vi "Interpret_LiDAR_Packet_Header.vi"(11 "Data in":u8[](array[numeric])) -> (2 "output cluster":T1 {"Ray Header Data"."Return Data Array"."Reflectance" format="%.6f %"; "Ray Header Data"."Return Data Array"."Range" format="%.4f M"; "Ray Header Data"."Return Data Array"."Existence Probability" format="%.4f %"; "Ray Header Data"."Elevation" format="%.6f"; "Ray Header Data"."Azimuth" format="%.6f"}, 3 "Remaining Data out":u8[](array[numeric]))   [LabVIEW 2018, in "LiDAR.lvlib" / "LiDAR.lvclass"]
uses:
  LiDAR.lvclass
  Controls/cls_Point_Cloud_Data.ctl
  Controls/cls_Point_Cloud_Packet_Header.ctl
  Controls/cls_Point_Cloud_Ray_Header.ctl
  Controls/cls_Point_Cloud_Return_Data.ctl
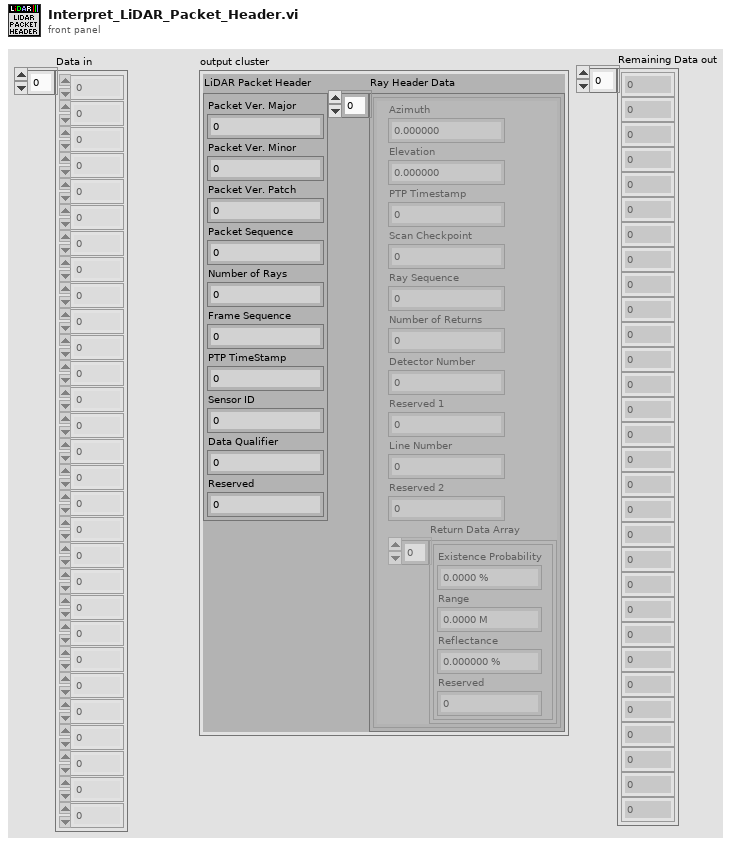
[diagram p1: front panel]
types:
  T1 = typedef "LiDAR.lvlib/LiDAR.lvclass/cls_Point_Cloud_Data.ctl" = cluster{"LiDAR Packet Header":T2, "Ray Header Data":T3[]}
  T2 = typedef "LiDAR.lvlib/LiDAR.lvclass/cls_Point_Cloud_Packet_Header.ctl" = cluster{"Packet Ver. Major":u8, "Packet Ver. Minor":u8, "Packet Ver. Patch":u8, "Packet Sequence":u8, "Number of Rays":u8, "Frame Sequence":u8, "PTP TimeStamp":u64, "Sensor ID":u8, "Data Qualifier":u8, "Reserved":u16}
  T3 = typedef "LiDAR.lvlib/LiDAR.lvclass/cls_Point_Cloud_Ray_Header.ctl" = cluster{"Azimuth":dbl, "Elevation":dbl, "PTP Timestamp":u32, "Scan Checkpoint":u8, "Ray Sequence":u8, "Number of Returns":u8, "Detector Number":u8, "Reserved 1":u8, "Line Number":u16, "Reserved 2":u32, "Return Data Array":T4[]}
  T4 = typedef "LiDAR.lvlib/LiDAR.lvclass/cls_Point_Cloud_Return_Data.ctl" = cluster{"Existence Probability":dbl, "Range":dbl, "Reflectance":dbl, "Reserved":u16}
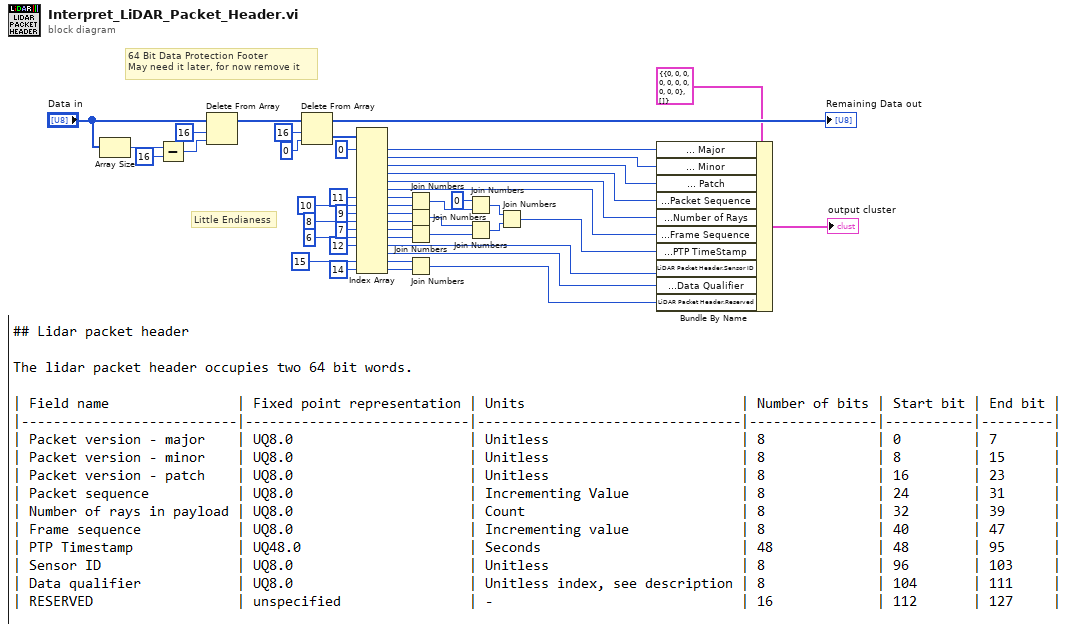
[diagram p0: block diagram]
diagram:
  # "Little Endianess"
  # "64 Bit Data Protection Footer\nMay need it later, for now remove it"
  n1 = Array Size(array="Data in") -> (size(s)=w13:i32)
  n2 = Subtract(x=w13, y=16) -> (x-y=w11:i32)
  n3 = Delete From Array(array="Data in", length=16, index=w11) -> (array with subset deleted=w14:u8[])  [unwired: 1 out]
  n4 = Delete From Array(array=w14, length=16, index=0) -> (deleted portion=w46:u8[], array with subset deleted=→"Remaining Data out":u8[])
  n5 = Index Array(array=w46, index #1=0 ("index"), index #7=11 ("index"), index #8=10 ("index"), index #9=9 ("index"), index #10=8 ("index"), index #11=7 ("index"), index #12=6 ("index"), index #13=12 ("index"), index #15=15 ("index"), index #16=14 ("index")) -> (element #1=w39:u8, element #2=w40:u8, element #3=w41:u8, element #4=w42:u8, element #5=w43:u8, element #6=w44:u8, element #7=w36:u8, element #8=w35:u8, element #9=w34:u8, element #10=w33:u8, element #11=w32:u8, element #12=w31:u8, element #13=w23:u8, element #14=w22:u8, element #15=w21:u8, element #16=w20:u8)  [unwired: 6 in]
  n6 = Join Numbers(hi=w36, lo=w35) -> ((hi.lo)=w28:u16)
  n7 = Join Numbers(hi=w34, lo=w33) -> ((hi.lo)=w29:u16)
  n8 = Join Numbers(hi=w32, lo=w31) -> ((hi.lo)=w30:u16)
  n9 = Join Numbers(hi=w21, lo=w20) -> ((hi.lo)=w19:u16)
  n10 = Join Numbers(hi=u16 0, lo=w28) -> ((hi.lo)=w25:u32)
  n11 = Join Numbers(hi=w29, lo=w30) -> ((hi.lo)=w26:u32)
  n12 = Join Numbers(hi=w25, lo=w26) -> ((hi.lo)=w24:u64)
  n13 = Bundle By Name(cluster=T1 {"LiDAR Packet Header"={"Packet Ver. Major"=0, "Packet Ver. Minor"=0, "Packet Ver. Patch"=0, "Packet Sequence"=0, "Number of Rays"=0, "Frame Sequence"=0, "PTP TimeStamp"=0, "Sensor ID"=0, "Data Qualifier"=0, "Reserved"=0}, "Ray Header Data"=[]} ("Point Cloud LiDAR Packet Header"), "LiDAR Packet Header.Packet Ver. Major"=w39, "LiDAR Packet Header.Packet Ver. Minor"=w40, "LiDAR Packet Header.Packet Ver. Patch"=w41, "LiDAR Packet Header.Packet Sequence"=w42, "LiDAR Packet Header.Number of Rays"=w43, "LiDAR Packet Header.Frame Sequence"=w44, "LiDAR Packet Header.PTP TimeStamp"=w24, "LiDAR Packet Header.Sensor ID"=w23, "LiDAR Packet Header.Data Qualifier"=w22, "LiDAR Packet Header.Reserved"=w19) -> (→"output cluster":T1)
